vi "Motor Wait.vi"(8 "error in":errorcluster, 11 "VISA resource name in":refnum<visa-resource-name>) -> (0 "error out":errorcluster, 3 "VISA resource name out":refnum<visa-resource-name>)   [LabVIEW 2015, in "JY-SPEX-TRIAX.lvlib"]
doc: "Waits until the motor busy flag is cleared."
uses:
  JY-SPEX-TRIAX.lvlib
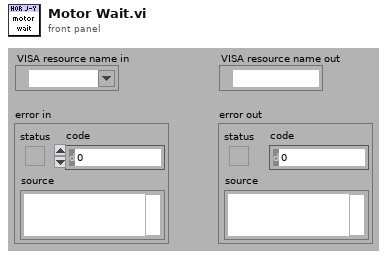
[diagram p1: front panel]
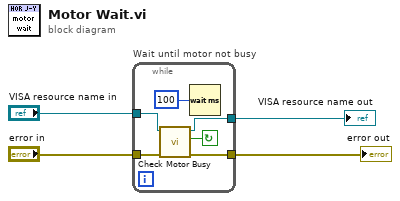
[diagram p0: block diagram]
diagram:
  n1 = while "Wait until motor not busy" {
    tunnel: "VISA resource name in" -> [w10]
    tunnel: [w9] -> w3
    tunnel: "error in" -> [w8]
    tunnel: [w7] -> w4
    stop <- w6 continue-if-true
    n2 = call "Check Motor Busy.vi"("error in (no error)"=w8, "VISA resource name"=w10) -> ("error out"=w7:errorcluster, "busy?"=w6:bool, "VISA resource name out"=w9:refnum<visa-resource-name>)  [unwired: 7 out]
    n3 = Wait (ms)(milliseconds to wait=u32 100) -> ()  [unwired: 1 out]
  }
  "error out" <- w4
  "VISA resource name out" <- w3
